vi "Create folders recursively.vi"(8 "error in (no error)":errorcluster, 11 "Path in":path) -> (0 "error out":errorcluster, 3 "Path out":path)   [LabVIEW 2015]
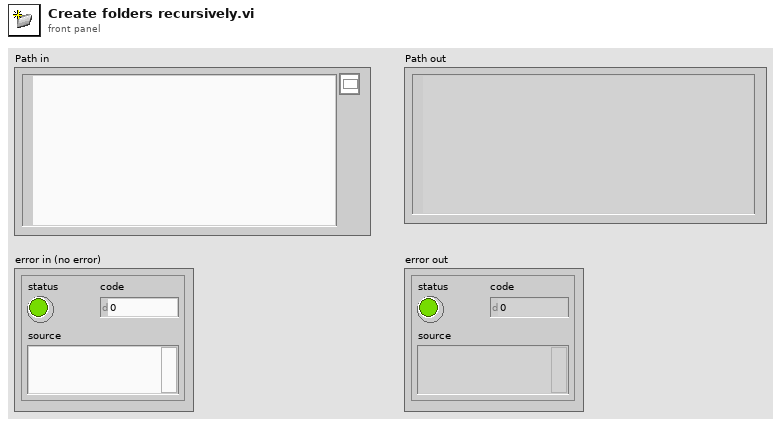
[diagram p1: front panel]
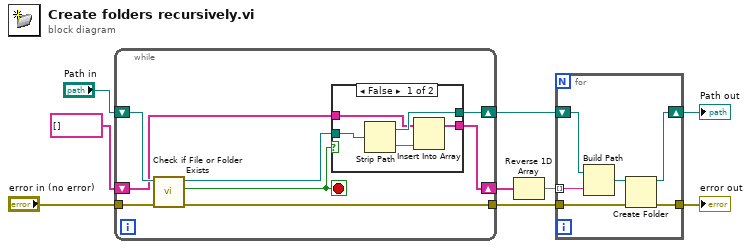
[diagram p0: block diagram]
diagram:
  n1 = while {
    shift-right: [w13] -> w5
    shift-left: string[] [] -> [w14]
    shift-right: [w15] -> w4
    shift-left: "Path in" -> [w16]
    tunnel: [w11] -> w6
    tunnel: "error in (no error)" -> [w10]
    stop <- w12 stop-if-true
    n2 = call <vilib>:"Check if File or Folder Exists.vi"("error in (no error)"=w10, "path"=w16) -> ("error out"=w11:errorcluster, "file or folder exists?"=w12:bool, "dup path"=w17:path)  [unwired: 7 in]
    n3 = case shown="False" w12 {
      tunnel: w17 -> [w22 w24]
      tunnel: [w21 w24] -> w15
      tunnel: w14 -> [w20 w23]
      tunnel: [w19 w23] -> w13
      frame False {
        n4 = Strip Path(path=w22) -> (stripped path=w21:path, name=w18:string)
        n5 = Insert Into Array(array=w20, new element=w18) -> (w19:string[])  [unwired: 1 in]
      }
      frame True {
      }
    }
  }
  n6 = Reverse 1D Array(array=w5) -> (reversed array=w1:string[])
  n7 = for {
    shift-right: [w27] -> w8
    shift-left: w4 -> [w30]
    tunnel: w1 -> [w29] mode=indexing
    tunnel: w6 -> [w26]
    tunnel: [w25] -> w9
    n8 = Build Path(base path=w30, name or relative path=w29) -> (appended path=w28:path)
    n9 = Create Folder(path (use dialog)=w28, error in=w26) -> (created path=w27:path, error out=w25:errorcluster)  [unwired: 1 in, 1 out]
  }
  "error out" <- w9
  "Path out" <- w8
